vi "Read Setting.vi"(0 "configuration file path":path, 3 "error in (no error)":errorcluster) -> (6 "file path":path, 7 "output cluster 2":T1, 9 "error out":errorcluster)   [LabVIEW 2023]
uses:
  <vilib>/Utility/config.llb/Read Key (String).vi
  <vilib>/Utility/config.llb/Read Key (U32).vi
  <vilib>/Utility/config.llb/Read Key (I32).vi
  <vilib>/Utility/config.llb/Read Key (Double).vi
  <vilib>/Utility/config.llb/Read Key (Path).vi
  <vilib>/Utility/config.llb/NI_LVConfig.lvlib
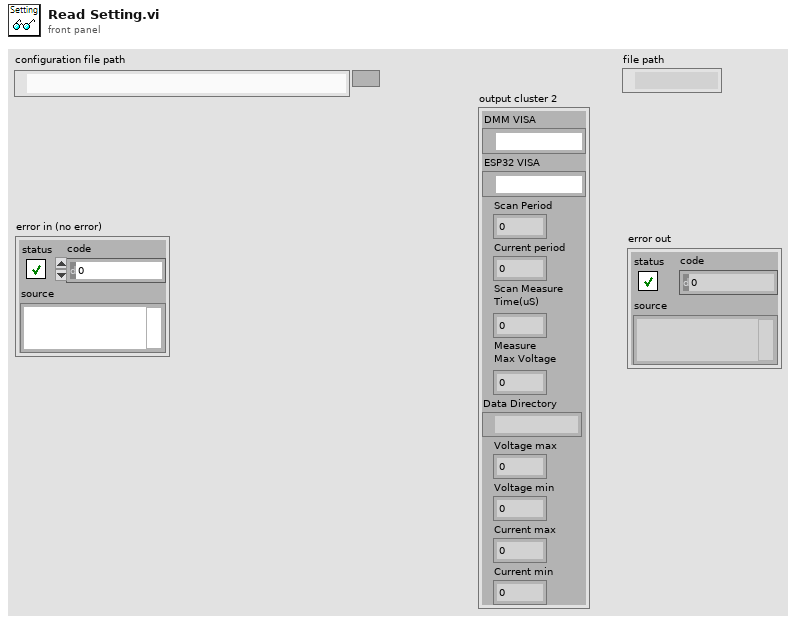
[diagram p1: front panel]
types:
  T1 = cluster{"DMM VISA":refnum<visa-resource-name>, "ESP32 VISA":refnum<visa-resource-name>, "Scan Period":u32, "Current period":u32, "Scan Measure\nTime(uS)":i32, "Measure\nMax Voltage":dbl, "Data Directory":path, "Voltage max":dbl, "Voltage min":dbl, "Current max":dbl, "Current min":dbl}
  T2 = typedef "NI_LVConfig.lvlib/Config Data RefNum.ctl" = refnum<k1>
  T3 = cluster{"value":string, "value":string, "value":u32, "value":u32, "value":i32, "value":dbl, "value":path, "value":dbl, "value":dbl, "value":dbl, "value":dbl}
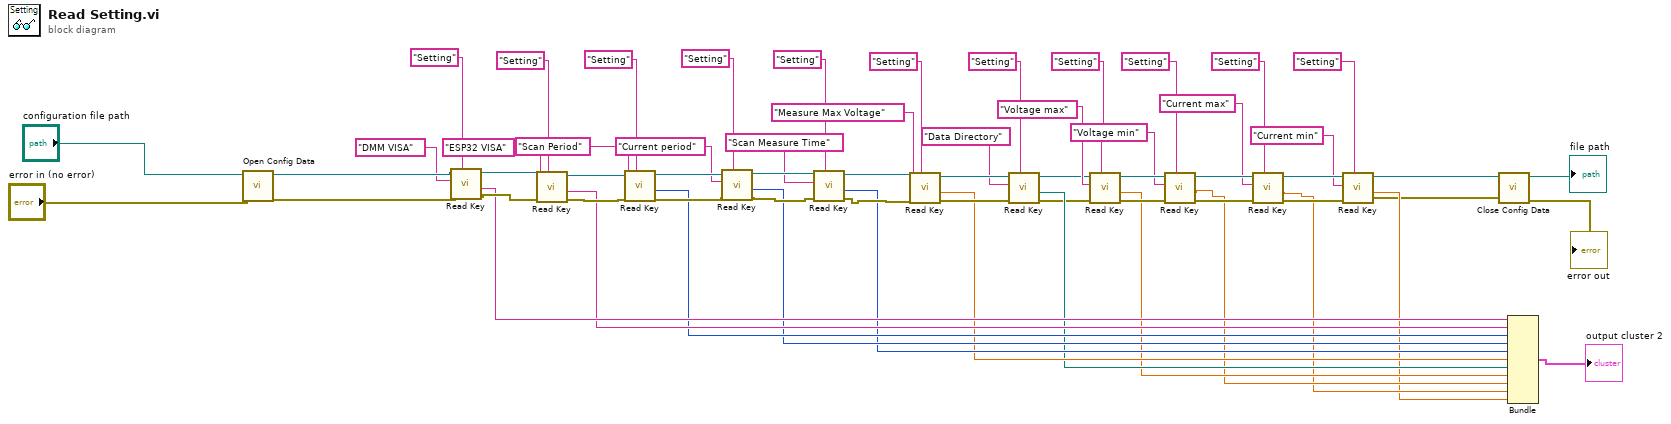
[diagram p0: block diagram]
diagram:
  n1 = call <vilib>:"Open Config Data.vi"("error in (no error)"="error in (no error)", "configuration file path"="configuration file path") -> ("error out"=w50:errorcluster, "refnum"=w51:T2)  [unwired: 7 in, 1 out]
  n2 = call-poly <vilib>:"Read Key.vi"("section"="Setting", "error in (no error)"=w50, "key"="DMM VISA", "refnum"=w51) -> ("error out"=w38:errorcluster, "value"=w30:string, "refnum out"=w49:T2)  [unwired: 4 in, 1 out]
  n3 = call-poly <vilib>:"Read Key.vi"("section"="Setting", "error in (no error)"=w38, "key"="ESP32 VISA", "refnum"=w49) -> ("error out"=w47:errorcluster, "value"=w29:string, "refnum out"=w48:T2)  [unwired: 4 in, 1 out]
  n4 = call-poly <vilib>:"Read Key.vi"("section"="Setting", "error in (no error)"=w47, "key"="Scan Period", "refnum"=w48) -> ("error out"=w45:errorcluster, "value"=w28:u32, "refnum out"=w46:T2)  [unwired: 4 in, 1 out]
  n5 = call-poly <vilib>:"Read Key.vi"("section"="Setting", "error in (no error)"=w45, "key"="Current period", "refnum"=w46) -> ("error out"=w43:errorcluster, "value"=w27:u32, "refnum out"=w44:T2)  [unwired: 4 in, 1 out]
  n6 = call-poly <vilib>:"Read Key.vi"("section"="Setting", "error in (no error)"=w43, "key"="Scan Measure Time", "refnum"=w44) -> ("error out"=w41:errorcluster, "value"=w26:i32, "refnum out"=w42:T2)  [unwired: 4 in, 1 out]
  n7 = call-poly <vilib>:"Read Key.vi"("section"="Setting", "error in (no error)"=w41, "key"="Measure Max Voltage", "refnum"=w42) -> ("error out"=w39:errorcluster, "value"=w25:dbl, "refnum out"=w40:T2)  [unwired: 4 in, 1 out]
  n8 = call-poly <vilib>:"Read Key.vi"("section"="Setting", "error in (no error)"=w39, "key"="Data Directory", "refnum"=w40) -> ("error out"=w8:errorcluster, "value"=w24:path, "refnum out"=w9:T2)  [unwired: 4 in, 1 out]
  n9 = call-poly <vilib>:"Read Key.vi"("section"="Setting", "error in (no error)"=w8, "key"="Voltage max", "refnum"=w9) -> ("error out"=w22:errorcluster, "value"=w7:dbl, "refnum out"=w23:T2)  [unwired: 4 in, 1 out]
  n10 = call-poly <vilib>:"Read Key.vi"("section"="Setting", "error in (no error)"=w22, "key"="Voltage min", "refnum"=w23) -> ("error out"=w20:errorcluster, "value"=w6:dbl, "refnum out"=w21:T2)  [unwired: 4 in, 1 out]
  n11 = call-poly <vilib>:"Read Key.vi"("section"="Setting", "error in (no error)"=w20, "key"="Current max", "refnum"=w21) -> ("error out"=w18:errorcluster, "value"=w5:dbl, "refnum out"=w19:T2)  [unwired: 4 in, 1 out]
  n12 = call-poly <vilib>:"Read Key.vi"("section"="Setting", "error in (no error)"=w18, "key"="Current min", "refnum"=w19) -> ("error out"=w1:errorcluster, "value"=w4:dbl, "refnum out"=w2:T2)  [unwired: 4 in, 1 out]
  n13 = call <vilib>:"Close Config Data.vi"("error in (no error)"=w1, "refnum"=w2) -> ("error out"=→"error out":errorcluster, "file path"=→"file path":path)  [unwired: 8 in]
  n14 = Bundle("value"=w30, "value"=w29, "value"=w28, "value"=w27, "value"=w26, "value"=w25, "value"=w24, "value"=w7, "value"=w6, "value"=w5, "value"=w4) -> (→"output cluster 2":T3)  [unwired: 1 in]
